vi "Pressure_Tapped_Cube.vi"(3 "Mode":T5, 5 "Traverse line In":T2 {"Carrier_2 Q (l/min)" format="%#.2f"; "Row Duration (mins)" format="%#.1f"; "Row No" min=0; "Trace Gas Concentration (%)" min=0.0 format="%#_4f"; "Carrier_1 Q (l/min)" format="%#.2f"; "Tunnel Speed" format="%#.2f"; "Start X" format="%#.2f"; "Start Y" format="%#.2f"; "Start Z" format="%#.2f"; "End X" format="%#.2f"; "End Y" format="%#.2f"; "End Z" format="%#.2f"; "Averaging time (min)" min=0.0 format="%#.2f"}) -> (0 "Error Message":string, 1 "Status":T1, 2 "Traverse line Out":T2 {"Carrier_2 Q (l/min)" format="%#.2f"; "Row Duration (mins)" format="%#.1f"; "Row No" min=0; "Trace Gas Concentration (%)" min=0.0 format="%#_4f"; "Carrier_1 Q (l/min)" format="%#.2f"; "Tunnel Speed" format="%#.2f"; "Start X" format="%#.2f"; "Start Y" format="%#.2f"; "Start Z" format="%#.2f"; "End X" format="%#.2f"; "End Y" format="%#.2f"; "End Z" format="%#.2f"; "Averaging time (min)" min=0.0 format="%#.2f"})   [LabVIEW 2014]
uses:
  Gen Trav/Traverse_cluster.ctl
  Gen Trav/Spacing.ctl
  Controls/Multi_run_mode.ctl
  Controls/User_Specific_mode.ctl
  Gen Trav/Multi_Run_Status.ctl
  Gen Trav/Trav_mode.ctl
  Controls/Setup.ctl
  Controls/Save_Data.ctl
  <vilib>/Analysis/baseanly.llb/Mean (DBL).vi
  Globals/Meas_global.vi
  <vilib>/Analysis/NI_AALBase.lvlib
panel:
  out "XY Graph":cluster{dbl[], dbl[]}(graph)
  out "Measurement No":i32
  in  "stop":bool
  # "X           Y            Z"
  # "Start"
  # "End"
  # "X           Y            Z"
  # "Start"
  # "End"
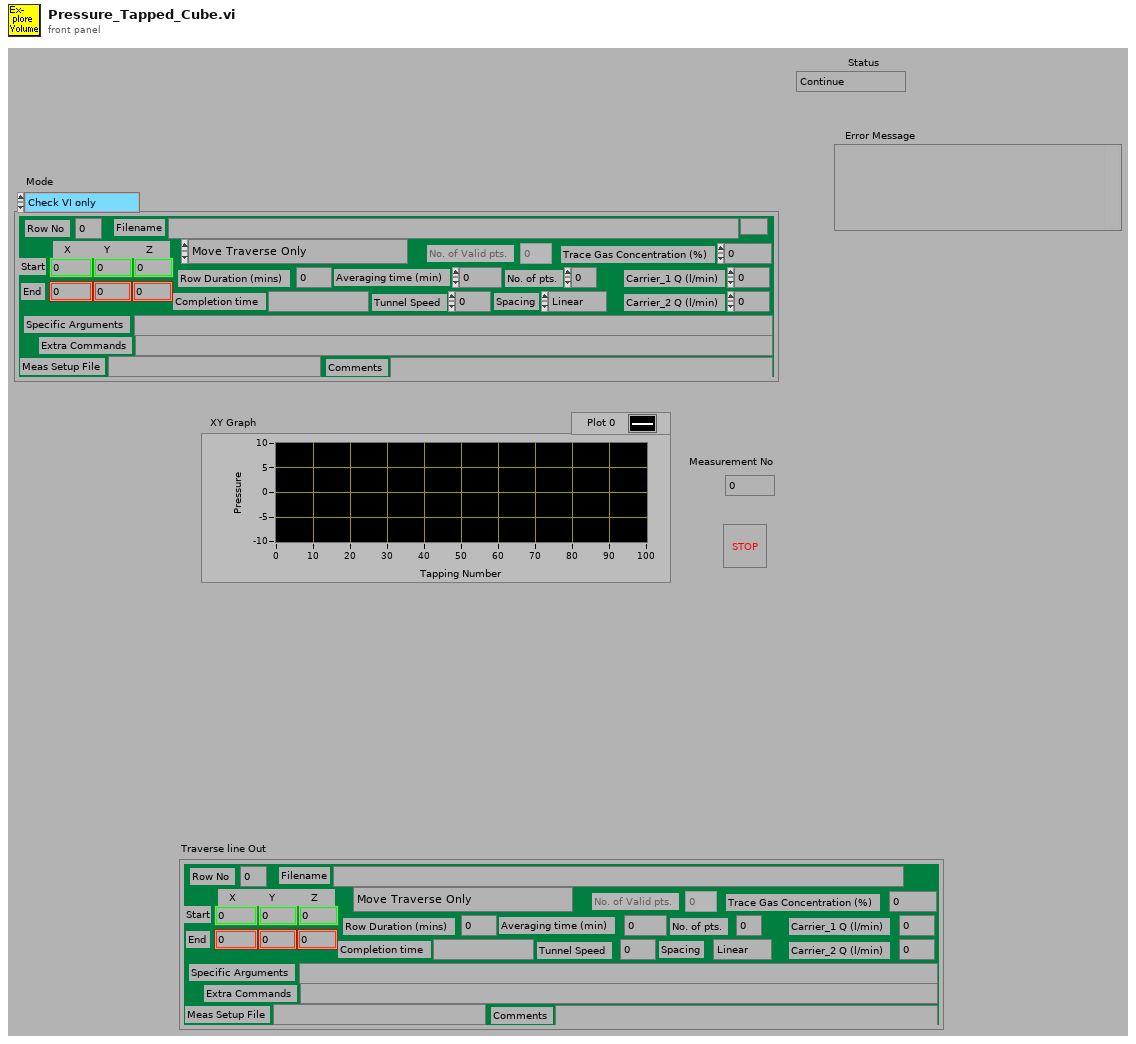
[diagram p1: front panel]
types:
  T1 = typedef "Multi_Run_Status.ctl" = enum16{"Continue", "Jump to Next Point", "Jump to Next Row", "Jump To Fall Back", "Terminate Run"}
  T2 = typedef "Traverse_cluster.ctl" = cluster{"Start X":sgl, "Start Y":sgl, "Start Z":sgl, "End X":sgl, "End Y":sgl, "End Z":sgl, "No. of pts.":i32, "Spacing":T3, "Filename":path, "Tunnel Speed":dbl, "Averaging time (min)":dbl, "Extra Commands":string, "Carrier_1 Q (l/min)":dbl, "Carrier_2 Q (l/min)":dbl, "Trace Gas Concentration (%)":dbl, "Specific Arguments":string, "Comments":string, "Row No":i32, "Row Type Selector":T4, "Completion time":string, "Row Duration (mins)":dbl, "No. of Valid pts.":i32, "Meas Setup File":string}
  T3 = typedef "Spacing.ctl" = enum16{"Linear", "Log", "Gauss", "Specified", "N/A"}
  T4 = typedef "Multi_run_mode.ctl" = enum16{"Move Traverse Only", "Set Tunnel Speed Only", "Set Source Only", "Set Measurement Conditions", "Single Measurement", "Vertical Profile", "Lateral Profile", "Longitudinal Profile", "Explore Volume", "Multi-Axis Profile", "Auto Calibrate", "Meas Fast FID Bkgnd", "Check Beam Power", "Scanning Valve Measurement", "Run VI Named:", "Set ADAM Ch", "Wait (minutes)", "Send Message", "Synchronize With:", "Fall Back to this Row", "Turn Off Row Repeating", "Blank Row", "Traverse 3D Volume"}
  T5 = typedef "User_Specific_mode.ctl" = enum16{"Check VI only", "Run VI"}
  T6 = typedef "Trav_mode.ctl" = enum16{"Move traverse", "Read traverse position", "Teach Position"}
  T7 = typedef "Save_Data.ctl" = enum16{"Save No Data", "Save Data"}
  T8 = typedef "Setup.ctl" = enum16{"Run Program", "Show Setup", "Save Current Setup", "Setup Front Panel"}
  T9 = typedef "Status_Cluster.ctl" = cluster{"Status":T1, "Error Type":string, "Error Description":string}
  T10 = typedef "Analysis_info_cluster.ctl" = cluster{"Colour":u32, "Inst type":T11, "Inst name":string, "Symbol":string, "Code name":string, "Extra Info":string, "Inst Array":T12, "Extra Titles":string[], "Extra Values":string[], "U":dbl, "u^2":dbl, "u^3":dbl, "u^4":dbl, "Skew_u":dbl, "Kurt_u":dbl, "Sd Error in Mean":dbl, "% u'/U":dbl, "X":dbl, "Y":dbl, "Z":dbl, "Timescale integral to 25%":dbl, "Sd Error in Variance":dbl, "Calib File":path, "Calib Constants":dbl[], "Output Position":bool, "Full Stats":bool, "Av Sampling Rate":dbl, "Av No of Samples":dbl, "Total Meas Time (s)":dbl, "ADAM Ch Name":string}
  T11 = typedef "Inst_type.ctl" = enum16{"Propeller anemometer", "Raw voltage", "Pressure Transducer", "Pitot-static tube", "Preston tube", "Hot wire", "Cross wire 1", "Cross wire 2", "Generic Linear", "Generic Polynomial", "Generic BackPoly", "Fast FID", "Thermocouple", "Cold wire", "Pulsed Wire", "LDA Vel", "LDA Tran time", "LDA Arr time", "Microphone"}
  T12 = typedef "Instrument_Array.ctl" = enum16{"PWA", "LDA", "Analogue"}
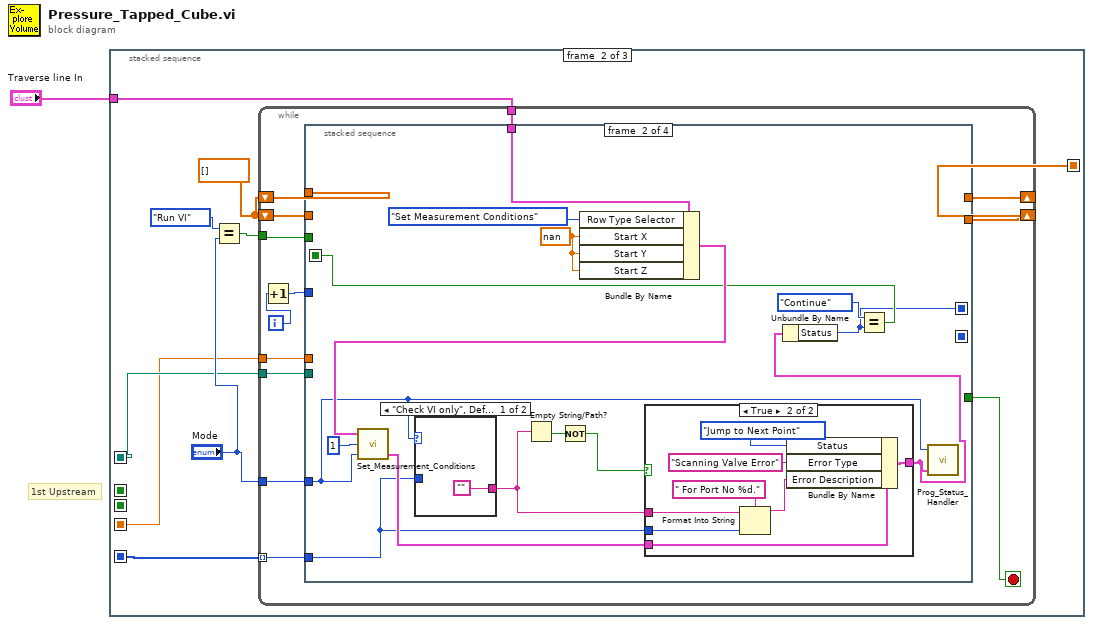
[diagram p0: block diagram]
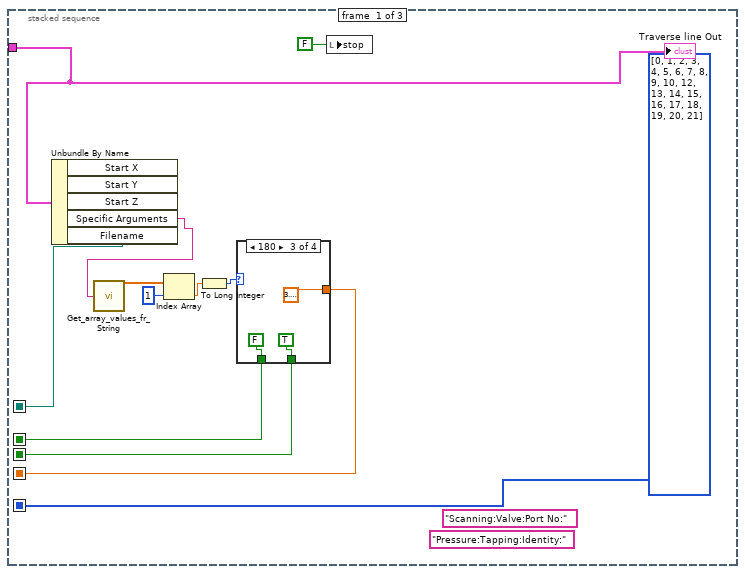
[diagram p2: hidden frame]
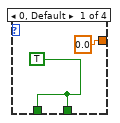
[diagram p3: hidden frame]
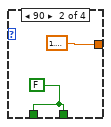
[diagram p4: hidden frame]
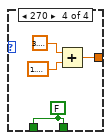
[diagram p5: hidden frame]
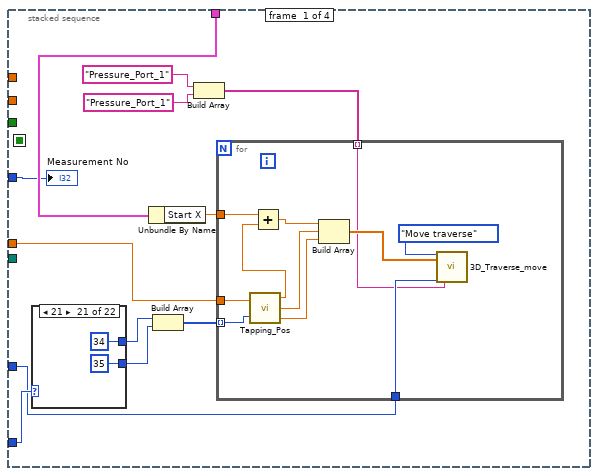
[diagram p6: hidden frame]
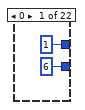
[diagram p7: hidden frame]
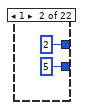
[diagram p8: hidden frame]
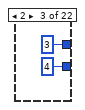
[diagram p9: hidden frame]
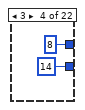
[diagram p10: hidden frame]
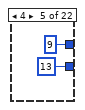
[diagram p11: hidden frame]
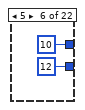
[diagram p12: hidden frame]
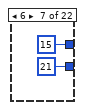
[diagram p13: hidden frame]
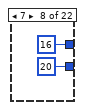
[diagram p14: hidden frame]
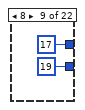
[diagram p15: hidden frame]
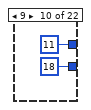
[diagram p16: hidden frame]
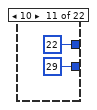
[diagram p17: hidden frame]
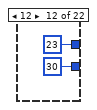
[diagram p18: hidden frame]
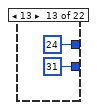
[diagram p19: hidden frame]
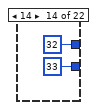
[diagram p20: hidden frame]
diagram:
  # "1st Upstream"
  n1 = stacked-sequence {
    seq-local: [w2 _ _] -> [_ w30 _]
    seq-local: [_ w29 _] -> [_ _ w222]
    seq-local: [w6 _ _] -> [_ _ w217]
    seq-local: [w4 _ _] -> [_ w26 _]
    seq-local: [w5 _ _] -> [_ _ w207]
    seq-local: [i32[] [0, 1, 2, 3, 4, 5, 6, 7, 8, 9, 10, 12, 13, 14, 15, 16, 17, 18, 19, 20, 21] _ _] -> [_ w25 _]
    tunnel: "Traverse line In" -> [w13 w27 _]
    frame #0 {
      (unwired) "Pressure:Tapping:Identity:"
      (unwired) "Scanning:Valve:Port No:"
      n2 = Unbundle By Name(w13) -> ("Specific Arguments"=w12:string, "Filename"=w2:path)  [unwired: 3 out]
      n3 = call "Get_array_values_fr_String.vi"("String Value"=w12) -> ("Numeric Array"=w10:dbl[])  [unwired: 1 out]
      n4 = Index Array(array=w10, index=1) -> (element=w8:dbl)
      n5 = To Long Integer(number=w8) -> (32bit integer=w7:i32)
      n6 = case shown="180" w7 {
        tunnel: [0.0 1.5707963267948966 3.141592653589793 w22] -> w4
        tunnel: [w14 w16 FALSE w21] -> w6
        tunnel: [w14 w16 TRUE w21] -> w5
        frame 0, Default {
          w14 = TRUE
        }
        frame 90 {
          w16 = FALSE
        }
        frame 180 {
        }
        frame 270 {
          w21 = FALSE
          n7 = Add(x=3.141592653589793, y=1.5707963267948966) -> (x+y=w22:dbl)
        }
      }
      n8 = local write "stop"(FALSE ("stop")) -> ()
      "Traverse line Out" <- w13
    }
    frame #1 {
      w28 = dbl[] []
      n9 = Equal?(x=User_Specific_mode."Run VI" ("Mode"), y="Mode") -> (x = y?=w31:bool)
      n10 = while {
        tunnel: "Mode" -> [w41]
        tunnel: w31 -> [w37]
        tunnel: w30 -> [w46]
        shift-right: [w44] -> w29
        shift-left: w28 -> [w45]
        shift-right: [w42] -> _
        shift-left: w28 -> [w43]
        tunnel: w27 -> [w40]
        tunnel: w26 -> [w39]
        tunnel: w25 -> [w34] mode=indexing
        i -> [w36]
        stop <- w38 stop-if-true
        n11 = Increment(x=w36) -> (x+1=w35:i32)
        n12 = stacked-sequence {
          seq-local: [_ w117 _ _] -> [_ _ w144 _]
          seq-local: [_ w116 _ _] -> [_ _ w145 _]
          seq-local: [_ _ w146 _] -> [_ _ _ w199]
          tunnel: w46 -> [_ _ w152 _]
          tunnel: w45 -> [_ _ w151 _]
          tunnel: [_ _ w150 _] -> w44
          tunnel: w43 -> [_ _ w149 _]
          tunnel: [_ _ w148 _] -> w42
          tunnel: w41 -> [w50 w120 _ _]
          tunnel: w40 -> [w58 w127 w147 _]
          tunnel: w35 -> [w52 _ _ w202]
          tunnel: w39 -> [w57 _ _ _]
          tunnel: [_ _ _ w200] -> w38
          tunnel: w37 -> [_ _ w143 _]
          tunnel: w34 -> [w51 w115 w141 _]
          frame #0 {
            n13 = case shown="21" w51 {
              tunnel: [1 2 3 8 9 10 15 16 17 11 22 23 24 32 36 37 39 41 26 28 34 -1] -> w56
              tunnel: [6 5 4 14 13 12 21 20 19 18 29 30 31 33 25 38 40 42 27 7 35 -1] -> w55
              frame 0 {
              }
              frame 1 {
              }
              frame 2 {
              }
              frame 3 {
              }
              frame 4 {
              }
              frame 5 {
              }
              frame 6 {
              }
              frame 7 {
              }
              frame 8 {
              }
              frame 9 {
              }
              frame 10 {
              }
              frame 12 {
              }
              frame 13 {
              }
              frame 14 {
              }
              frame 15 {
              }
              frame 16 {
              }
              frame 17 {
              }
              frame 18 {
              }
              frame 19 {
              }
              frame 20 {
              }
              frame 21 {
              }
              frame 22, Default {
              }
            }
            n14 = Unbundle By Name(w58) -> ("Start X"=w53:sgl)
            n15 = Build Array(w56, w55) -> (w54:i32[])
            n16 = Build Array("Pressure_Port_1", "Pressure_Port_1") -> (w47:string[])
            n17 = for {
              tunnel: w57 -> [w113]
              tunnel: w54 -> [w112] mode=indexing
              tunnel: w53 -> [w111]
              tunnel: w50 -> [w104]
              tunnel: w47 -> [w103] mode=indexing
              n18 = call "Tapping_Pos.vi"("Orientation"=w113, "Tapping Number"=w112) -> ("X"=w110:sgl, "Y"=w107:sgl, "Z"=w108:sgl)
              n19 = Add(x=w111, y=w110) -> (x+y=w109:sgl)
              n20 = Build Array(w109, w107, w108) -> (w106:sgl[])
              n21 = call "3D_Traverse_move.vi"("Mode"=Trav_mode."Move traverse", "Position"=w106, "Simulate/Run"=w104, "Traverse name"=w103) -> ()  [unwired: 13 in, 3 out]
            }
            "Measurement No" <- w52
          }
          frame #1 {
            w114 = sgl nan ("Start X")
            n22 = case shown="\"Check VI only\", Default" w120 {
              tunnel: w115 -> [_ w131]
              tunnel: ["" w130] -> w121
              frame "Check VI only", Default {
              }
              frame "Run VI" {
                n23 = call "ScaniValve_client.vi"("Port Number"=w131) -> ("Error String"=w130:string)  [unwired: 2 out]
              }
            }
            n24 = Empty String/Path?(string/path=w121) -> (empty?=w124:bool)
            n25 = Not(x=w124) -> (.not. x?=w123:bool)
            n26 = Bundle By Name(cluster=w127, "Row Type Selector"=Multi_run_mode."Set Measurement Conditions", "Start X"=w114, "Start Y"=w114, "Start Z"=w114) -> (w125:T2)
            n27 = call "Set_Measurement_Conditions.vi"("Simulate/Run"=w120, "Currently on Point"=1, "Traverse line"=w125) -> ("Status Cluster"=w122:T9)  [unwired: 2 out]
            n28 = case shown="True" w123 {
              tunnel: w122 -> [w132 w140]
              tunnel: [w132 w137] -> w118
              tunnel: w121 -> [_ w134]
              tunnel: w115 -> [_ w133]
              frame False {
              }
              frame True {
                n29 = Format Into String(format string=" For Port No %d." ("Format String"), initial string=w134, w133) -> (resulting string=w135:string)  [unwired: 1 in, 1 out]
                n30 = Bundle By Name(cluster=w140, "Status"=Multi_Run_Status."Jump to Next Point", "Error Type"="Scanning Valve Error" ("t"), "Error Description"=w135) -> (w137:T9)
              }
            }
            n31 = Unbundle By Name(w118) -> ("Status"=w116:T1)
            n32 = Equal?(x=Multi_Run_Status."Continue" ("Status"), y=w116) -> (x = y?=w117:bool)
            n33 = call "Prog_Status_Handler.vi"("Status Cluster"=w118, "Simulate/Run"=w120) -> ()  [unwired: 2 out]
          }
          frame #2 {
            n34 = And(x=w143, y=w144) -> (x .and. y?=w142:bool)
            n35 = case shown="True" w142 {
              tunnel: [w153 w163] -> w146
              tunnel: w152 -> [_ w162]
              tunnel: w151 -> [w155 w161]
              tunnel: [w155 w160] -> w150
              tunnel: w149 -> [w154 w159]
              tunnel: [w154 w158] -> w148
              tunnel: w147 -> [_ w157]
              tunnel: w141 -> [_ w156]
              tunnel: w145 -> [w153 _]
              frame False {
                (unwired) FALSE ("stop")
              }
              frame True {
                n36 = stacked-sequence {
                  seq-local: [_ w174 _] -> [_ _ w190]
                  tunnel: [w166 _ _] -> w163
                  tunnel: w162 -> [w165 _ _]
                  tunnel: w161 -> [_ w175 _]
                  tunnel: [_ w174 _] -> w160
                  tunnel: w159 -> [_ _ w195]
                  tunnel: [_ _ w193] -> w158
                  tunnel: w157 -> [w164 _ _]
                  tunnel: w156 -> [_ _ w188]
                  frame #0 {
                    w169 = TRUE  # Open Front Panel
                    w171 = FALSE  # Remote control
                    n37 = Unbundle By Name(w164) -> ("Averaging time (min)"=w170:dbl)
                    n38 = call "Code_to_run.vi"("Open Front Panel"=w169, "setup"=Setup."Run Program", "Remote control"=w171, "File"=Save_Data."Save Data", "Results Filename"=w165, "Averaging time (min)"=w170) -> ("Status"=w166:T1)  [unwired: 5 in, 4 out]
                  }
                  frame #1 {
                    n39 = global read "Meas_global.vi" "Analysis Info cluster"() -> (w173:T10[])
                    n40 = Array Size(array=w173) -> (size(s)=w172:i32)
                    n41 = while {
                      tunnel: w173 -> [w187] mode=indexing
                      tunnel: [w185] -> _ mode=indexing
                      tunnel: [w186] -> w176
                      tunnel: w172 -> [w182]
                      i -> [w183]
                      stop <- w177 continue-if-true
                      n42 = Decrement(x=w182) -> (x-1=w181:i32)
                      n43 = Unbundle By Name(w187) -> ("Inst name"=w185:string, "U"=w186:dbl)
                      n44 = Match Pattern(string=w185, regular expression="Mano") -> (offset past match=w180:i32)  [unwired: 4 out]
                      n45 = Less?(x=w183, y=w181) -> (x < y?=w178:bool)
                      n46 = Less Than 0?(x=w180) -> (x < 0?=w179:bool)
                      n47 = And(x=w179, y=w178) -> (x .and. y?=w177:bool)
                    }
                    n48 = Build Array (concatenate)(w175, w176) -> (w174:dbl[])
                  }
                  frame #2 {
                    n49 = Build Array (concatenate)(w195, w188) -> (w193:dbl[])
                    n50 = call "Sort_Array_Indicies.vi"("unsorted array"=w193) -> ("sorted array"=w192:dbl[], "Sort Index"=w191:i32[])
                    n51 = for {
                      tunnel: w191 -> [w198] mode=indexing
                      tunnel: w190 -> [w197]
                      tunnel: [w196] -> w189 mode=indexing
                      n52 = Index Array(array=w197, index=w198) -> (element=w196:dbl)
                    }
                    n53 = Bundle("sorted array"=w192, w189) -> (→"XY Graph":cluster{"sorted array":dbl[], dbl[]})  [unwired: 1 out]
                  }
                }
              }
            }
          }
          frame #3 {
            n54 = Greater?(x=w199, y=Multi_Run_Status."Jump to Next Point" ("Status")) -> (0:w205:bool)
            n55 = Greater Or Equal?(x=w202, y=21.0) -> (x >= y?=w204:bool)
            n56 = Compound Arithmetic op=OR("stop", w205, w204) -> (w200:bool)
            "Status" <- w199
          }
        }
      }
    }
    frame #2 {
      n57 = Split 1D Array(array=w222, index=21) -> (first subarray=w220:dbl[], second subarray=w216:dbl[])
      n58 = Array Size(array=w216) -> (size(s)=w215:i32)
      n59 = call-poly <vilib>:"Mean.vi"("X"=w220) -> ("mean"=w219:dbl)  [unwired: 1 out]
      n60 = call-poly <vilib>:"Mean.vi"("X"=w216) -> ("mean"=w218:dbl)  [unwired: 1 out]
      n61 = Greater?(x=w215, y=19) -> (0:w208:bool)
      n62 = case shown="False" w217 {
        tunnel: w219 -> [w225 w228]
        tunnel: w218 -> [w224 w227]
        tunnel: [w223 w226] -> w213
        frame False {
          n63 = Greater?(x=w225, y=w224) -> (0:w223:bool)
        }
        frame True {
          n64 = Less?(x=w228, y=w227) -> (x < y?=w226:bool)
        }
      }
      n65 = Compound Arithmetic op=AND(w213, w208, w207) -> (w212:bool)
      n66 = Select(t="The Pressures on the upstream face are lower than the downstream face.\nMaybe you have incorrectly entered the orientation of the cube via the second specific argument.", s=w212, f="") -> (s? t:f=→"Error Message":string)
    }
  }
